vi "Write Current_Share.vi"(8 "error in":errorcluster, 10 "Current_Sharing":bool, 11 "6032A in":refnum<class "6032A.lvclass">) -> (0 "error out":errorcluster, 3 "6032A out":refnum<class "6032A.lvclass">)   [LabVIEW 2019, in "6032A.lvlib" / "6032A.lvclass"]
uses:
  Library/6032A.lvclass
  C:/Users/Public/Documents/Development/builds/Instruments/PowerSupply.lvlibp/Library/PowerSupply.lvclass
  builds/Instruments/PowerSupply.lvlibp/Accessors/Settings/Unsupported Function.vi
  builds/Instruments/PowerSupply.lvlibp/Library/PowerSupply.lvclass
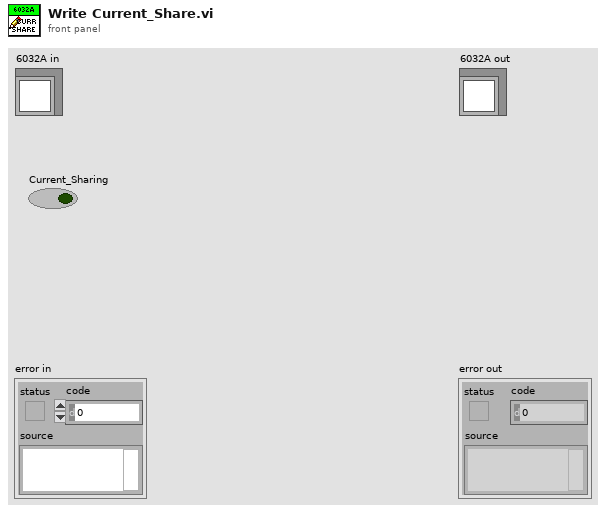
[diagram p1: front panel]
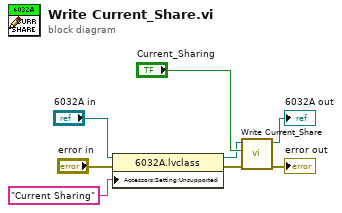
[diagram p0: block diagram]
diagram:
  n1 = property class="6032A.lvclass"(reference="6032A in", error in="error in", "Accessors:Setting:Unsupported"="Current Sharing" ("Supply:Warning:Unsupported")) -> (reference out=w3:refnum<class "6032A.lvclass">, error out=w2:errorcluster)
  n2 = call-parent "Write Current_Share.vi"("error in"=w2, "Current_Sharing"="Current_Sharing", "PowerSupply in"=w3) -> ("error out"=→"error out":errorcluster, "PowerSupply out"=→"6032A out":refnum<class "6032A.lvclass">)  [unwired: 7 in]
